vi "Shoot3.vi"(11 "Elapsed":dbl) -> (3 "All Driver Commands":T1)   [LabVIEW 2012]
uses:
  All_Commands.ctl
  Cirular Shooter/circular_shooter_commands.ctl
  Climber/Climber_Commands.ctl
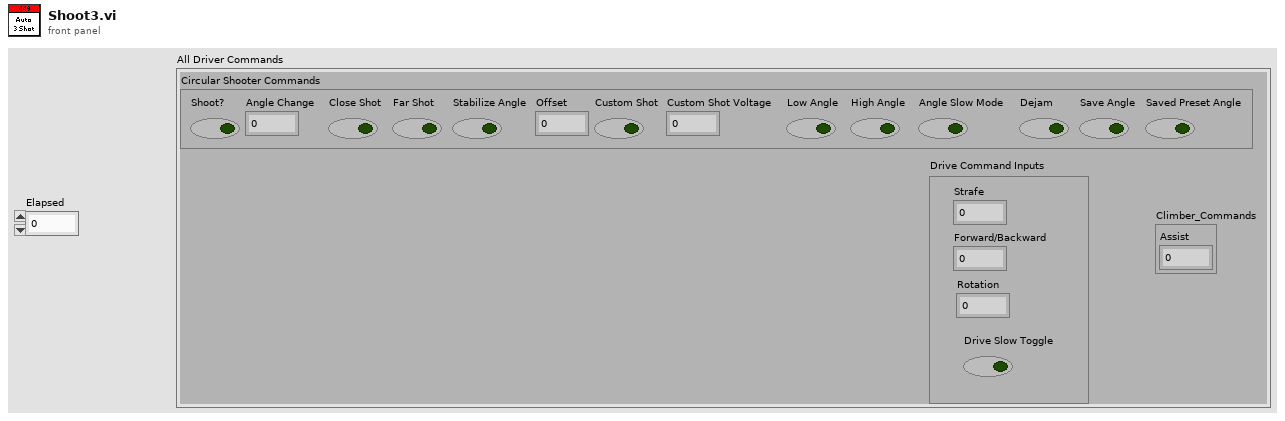
[diagram p1: front panel]
types:
  T1 = typedef "All_Commands.ctl" = cluster{"Circular Shooter Commands":T2, "Drive Command Inputs":cluster{"Strafe":dbl, "Forward/Backward":dbl, "Rotation":dbl, "Drive Slow Toggle":bool}, "Climber_Commands":T3}
  T2 = typedef "circular_shooter_commands.ctl" = cluster{"Shoot?":bool, "Angle Change":dbl, "Close Shot":bool, "Far Shot":bool, "Stabilize Angle ":bool, "Offset":dbl, "Custom Shot":bool, "Custom Shot Voltage":dbl, "Low Angle":bool, "High Angle":bool, "Angle Slow Mode":bool, "Dejam":bool, "Save Angle":bool, "Saved Preset Angle":bool}
  T3 = typedef "Climber_Commands.ctl" = cluster{"Assist":dbl}
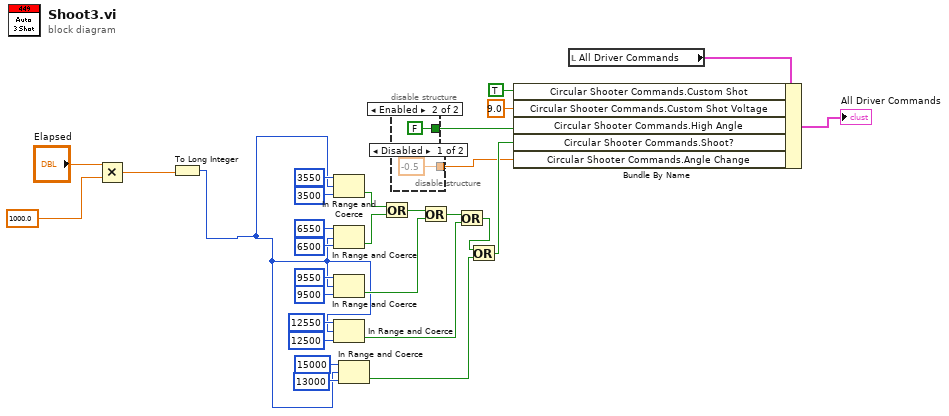
[diagram p0: block diagram]
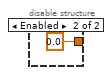
[diagram p2: hidden frame]
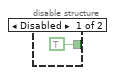
[diagram p3: hidden frame]
diagram:
  n1 = Multiply(x="Elapsed", y=1000.0) -> (x*y=w8:dbl)
  n2 = To Long Integer(number=w8) -> (32bit integer=w5:i32)
  n3 = In Range and Coerce(upper limit=u32 3550 ("y"), x=w5, lower limit=u32 3500) -> (In Range?=w19:bool)  [unwired: 1 out]
  n4 = In Range and Coerce(upper limit=u32 6550, x=w5, lower limit=u32 6500) -> (In Range?=w17:bool)  [unwired: 1 out]
  n5 = In Range and Coerce(upper limit=u32 9550, x=w5, lower limit=u32 9500) -> (In Range?=w16:bool)  [unwired: 1 out]
  n6 = In Range and Coerce(upper limit=u32 12550, x=w5, lower limit=u32 12500) -> (In Range?=w11:bool)  [unwired: 1 out]
  n7 = In Range and Coerce(upper limit=15000, x=w5, lower limit=13000) -> (In Range?=w4:bool)  [unwired: 1 out]
  n8 = Or(x=w19, y=w17) -> (x .or. y?=w18:bool)
  n9 = disable-structure shown="Enabled" {
    disable-tunnel: [TRUE FALSE] -> w25
    frame Disabled {
    }
    frame Enabled {
    }
  }
  n10 = disable-structure shown="Disabled" {
    disable-tunnel: [-0.5 ("Circular Shooter Commands.Angle Change") 0.0 ("Circular Shooter Commands.Angle Change")] -> w1
    frame Disabled {
    }
    frame Enabled {
    }
  }
  n11 = Or(x=w18, y=w16) -> (x .or. y?=w15:bool)
  n12 = Or(x=w15, y=w11) -> (x .or. y?=w3:bool)
  n13 = Or(x=w3, y=w4) -> (x .or. y?=w2:bool)
  n14 = local read "All Driver Commands"() -> (w28:T1)
  n15 = Bundle By Name(cluster=w28, "Circular Shooter Commands.Custom Shot"=TRUE, "Circular Shooter Commands.Custom Shot Voltage"=9.0, "Circular Shooter Commands.High Angle"=w25, "Circular Shooter Commands.Shoot?"=w2, "Circular Shooter Commands.Angle Change"=w1) -> (→"All Driver Commands":T1)
